vi "sincosSGL.vi"(5 "x":sgl) -> (6 "sinx":sgl, 8 "cosx":sgl)   [LabVIEW 2015]
doc: "x is in units of pi radians."
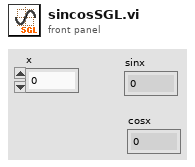
[diagram p1: front panel]
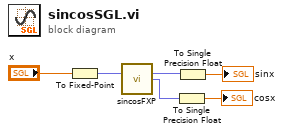
[diagram p0: block diagram]
diagram:
  n1 = To Fixed-Point(number="x") -> (fixed-point=w5:fxp<+/-,16,1>)  [unwired: 1 in]
  n2 = call "sincosFXP.vi"("x"=w5) -> ("sinx"=w4:fxp<+/-,16,2>, "cosx"=w3:fxp<+/-,16,2>)  [unwired: 13 in]
  n3 = To Single Precision Float(number=w3) -> (single precision float=→"cosx":sgl)
  n4 = To Single Precision Float(number=w4) -> (single precision float=→"sinx":sgl)
